vi "PCO_GetCompressionMode.vi"(8 "error in (no error)":errorcluster {"code" format="%x"}, 11 "ph":u64) -> (0 "error out":errorcluster {"code" format="%x"}, 1 "wCompressionMode":u16, 2 "ErrorMessage":i32 format="%x", 3 "ph out":u64)   [LabVIEW 2019, in "SDK.lvlib" / "StorageControl.lvlib"]
doc: "<b>Description:</b>\nGets the ram compression mode of the camera. Please check camera descriptor 3 for availability.\n\n<b>Supported camera type:</b>\npco.dimax, pco.1200, pco.1600, pco.2000, pco.4000\n\n<b>Descriptor dependency:</b>\ndwGeneralCapsDESC3"
uses:
  StorageControl.lvlib
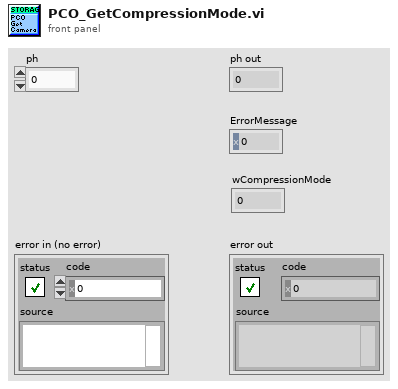
[diagram p1: front panel]
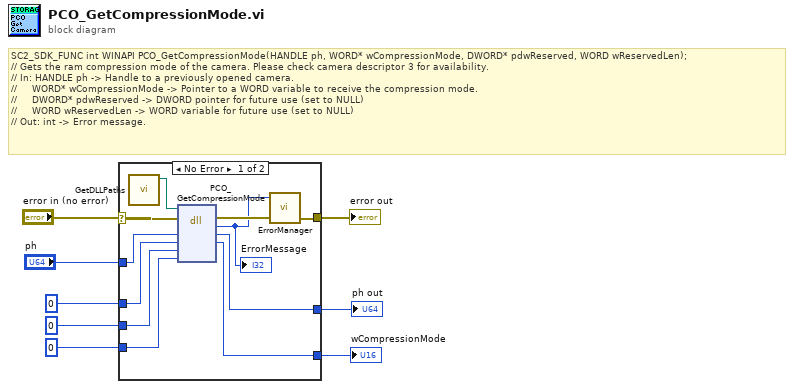
[diagram p0: block diagram]
diagram:
  # "SC2_SDK_FUNC int WINAPI PCO_GetCompressionMode(HANDLE ph, WORD* wCompressionMode, DWORD* pdwReserved, WORD wReservedLen);\n// Gets the ram compression mode of the camera. Please check camera descriptor 3 for availability.\n// In: HANDLE ph -> Handle to a previously opened camera.\n//     WORD* wCompressionMode -> Pointer to a WORD variable to receive the compression mode.\n//     DWORD* pdwReserved -> DWORD pointer for future use (set to NULL)\n//     WORD wReservedLen -> WORD variable for future use (set to NULL)\n// Out: int -> Error message."
  n1 = case shown="No Error" "error in (no error)" {
    selector: "error in (no error)" -> [w16 w22]
    tunnel: "ph" -> [w19 w21]
    tunnel: [w18 w21] -> w7
    tunnel: [w14 w22] -> w6
    tunnel: [w17 w20] -> w5
    tunnel: u16 0 -> [w11 w20]
    tunnel: u32 0 -> [w10 _]
    tunnel: u16 0 -> [w9 _]
    frame No Error {
      n2 = call "GetDLLPaths.vi"() -> ("SC2_Cam_Path"=w12:path)  [unwired: 8 in, 3 out]
      n3 = dll-call lib="?" fn="PCO_GetCompressionMode"(path in=w12, error in=w16, "ph"=w19, "wCompressionMode"=w11, "pdwReserved"=w10, "wReservedLen"=w9) -> (error out=w15:errorcluster, "return type"=w13:i32, "ph"=w18:u64, "wCompressionMode"=w17:u16)  [unwired: 3 in, 1 out]
      "ErrorMessage" <- w13
      n4 = call "ErrorManager.vi"("error in (no error)"=w15, "error code"=w13) -> ("error out"=w14:errorcluster)  [unwired: 2 in, 1 out]
    }
    frame Error {
    }
  }
  "ph out" <- w7
  "error out" <- w6
  "wCompressionMode" <- w5
